vi "nearCamClose.vi"(1 "错误输入（无错误）":errorcluster) -> (0 "错误输出":errorcluster)   [LabVIEW 2018]
uses:
  VsyCam.dll
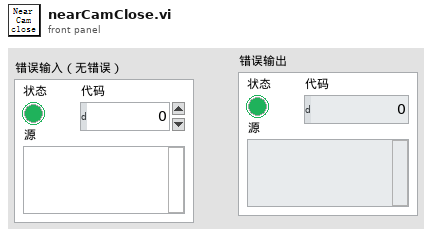
[diagram p1: front panel]
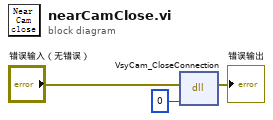
[diagram p0: block diagram]
diagram:
  n1 = dll-call lib="PTH2?abs D做的项目航天测量软件相机\nVsyCam.dll" fn="VsyCam_CloseConnection"(error in="错误输入（无错误）", "sockFd"=0) -> (error out=→"错误输出":errorcluster)  [unwired: 4 in, 1 out]
